vi "Save_to_Project.vi"(8 "error in (no error)":errorcluster, 9 "index in":string, 10 "buildObject":T1, 11 "Class in":refnum<class "IB_Source_Container.lvclass">) -> (0 "error out":errorcluster, 1 "index out":string, 2 "buildObject out":T1, 3 "Class out":refnum<class "IB_Source_Container.lvclass">, 5 "saved?":bool)   [LabVIEW 2020, in "IB_Source_Container.lvclass"]
uses:
  <vilib>/AppBuilder/IB_Classes/Source/Container/IB_Source_Container.lvclass
  <vilib>/AppBuilder/IB_Classes/Source/Container/IB_Source_Container.lvclass/IB_Source_Container.ctl
  <vilib>/AppBuilder/IB_Classes/Source/IB_Source.lvclass
  <vilib>/AppBuilder/IB_Classes/Source/File/CtrFile/IB_CtrFile.lvclass
  <resource>/Framework/Providers/API/ItemRef.ctl
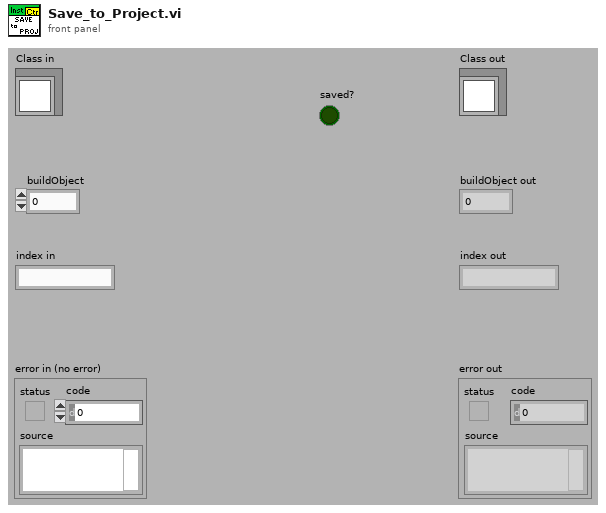
[diagram p1: front panel]
types:
  T1 = typedef "ItemRef.ctl" = u64
  T2 = typedef "IB_CtrFile.ctl" = cluster{"parentTag":string, "force save?":bool}
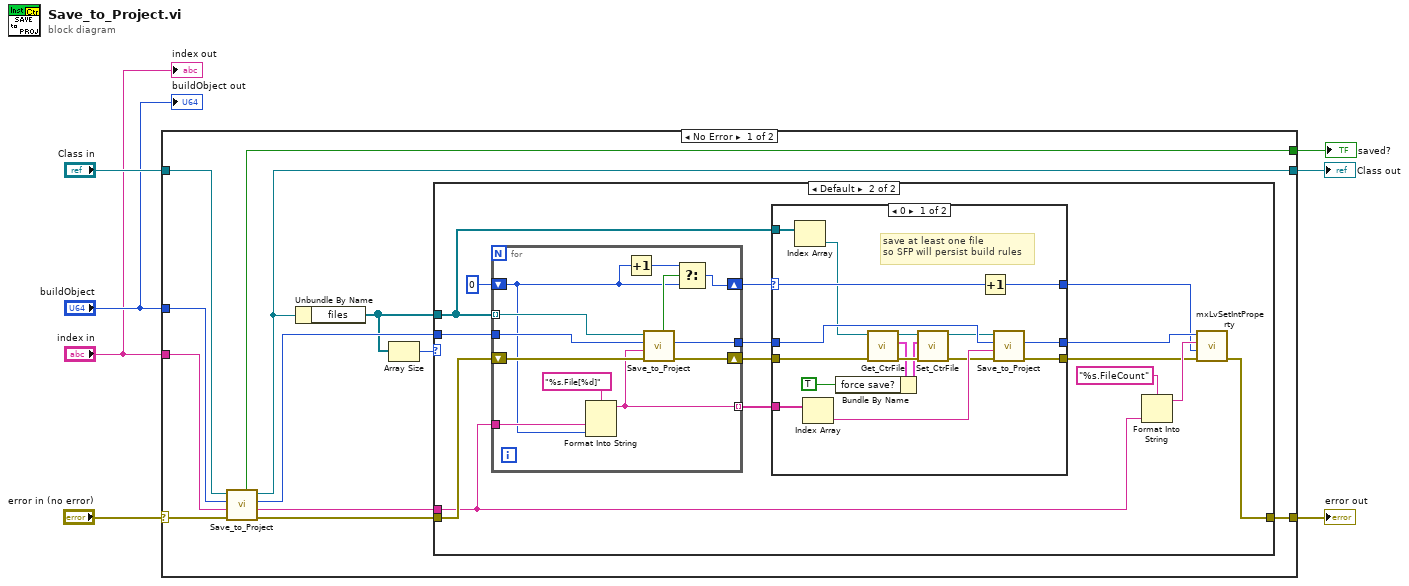
[diagram p0: block diagram]
diagram:
  n1 = case shown="No Error" "error in (no error)" {
    selector: "error in (no error)" -> [w16 w69]
    tunnel: [w9 w69] -> w7
    tunnel: [w15 w68] -> w6
    tunnel: "index in" -> [w19 _]
    tunnel: "buildObject" -> [w18 _]
    tunnel: "Class in" -> [w17 w68]
    tunnel: [w8 _] -> w1
    frame No Error {
      n2 = call-parent "Save_to_Project.vi"("error in (no error)"=w16, "index in"=w19, "buildObject"=w18, "Class in"=w17) -> ("error out"=w10:errorcluster, "index out"=w12:string, "buildObject out"=w14:T1, "Class out"=w15:refnum<class "IB_Source_Container.lvclass">, "saved?"=w8:bool)  [unwired: 3 out]
      n3 = Unbundle By Name(w15) -> ("files"=w13:refnum<class "IB_CtrFile.lvclass">[])
      n4 = Array Size(array=w13) -> (size(s)=w11:i32)
      n5 = case shown="Default" w11 {
        tunnel: w14 -> [_ w35]
        tunnel: w13 -> [_ w23]
        tunnel: w12 -> [_ w22]
        tunnel: w10 -> [w20 w33]
        tunnel: [w20 w27] -> w9
        frame 0 {
        }
        frame Default {
          n6 = for {
            tunnel: w23 -> [w67] mode=indexing
            tunnel: w35 -> [w66]
            tunnel: w22 -> [w64]
            shift-right: [w63] -> w34
            shift-left: w33 -> [w62]
            tunnel: [w61] -> w26
            shift-right: [w59] -> w31
            shift-left: 0 -> [w57]
            tunnel: [w56] -> w21 mode=indexing
            n7 = Format Into String(format string="%s.File[%d]", w64, w57) -> (resulting string=w56:string)  [unwired: 2 in, 1 out]
            n8 = Increment(x=w57) -> (x+1=w60:i32)
            n9 = call-dynamic "Save_to_Project.vi"("error in (no error)"=w62, "index in"=w56, "buildObject"=w66, "Class in"=w67) -> ("error out"=w63:errorcluster, "buildObject out"=w61:T1, "saved?"=w58:bool)  [unwired: 5 out]
            n10 = Select(t=w60, s=w58, f=w57) -> (s? t:f=w59:i32)
          }
          n11 = case shown="0" w31 {
            selector: w31 -> [w51 w53]
            tunnel: w34 -> [w40 w55]
            tunnel: [w52 w55] -> w28
            tunnel: w26 -> [w50 w54]
            tunnel: [w49 w54] -> w25
            tunnel: [w48 w53] -> w24
            tunnel: w23 -> [w47 _]
            tunnel: w21 -> [w46 _]
            frame 0 {
              # "save at least one file\nso SFP will persist build rules"
              n12 = Index Array(array=w47) -> (element=w42:refnum<class "IB_CtrFile.lvclass">)  [unwired: 1 in]
              n13 = Index Array(array=w46) -> (element=w45:string)  [unwired: 1 in]
              n14 = call <vilib>:"Get_CtrFile.vi"("error in (no error)"=w40, "IB_CtrFile in"=w42) -> ("error out"=w44:errorcluster, "parentTag"=w38:T2, "IB_CtrFile out"=w43:refnum<class "IB_CtrFile.lvclass">)  [unwired: 7 out]
              n15 = Bundle By Name(cluster=w38, "force save?"=TRUE) -> (w37:T2)
              n16 = call <vilib>:"Set_CtrFile.vi"("error in (no error)"=w44, "parentTag"=w37, "IB_CtrFile in"=w43) -> ("error out"=w39:errorcluster, "IB_CtrFile out"=w41:refnum<class "IB_CtrFile.lvclass">)  [unwired: 7 out]
              n17 = Increment(x=w51) -> (x+1=w48:i32)
              n18 = call-dynamic "Save_to_Project.vi"("error in (no error)"=w39, "index in"=w45, "buildObject"=w50, "Class in"=w41) -> ("error out"=w52:errorcluster, "buildObject out"=w49:T1)  [unwired: 6 out]
            }
            frame Default {
            }
          }
          n19 = Format Into String(format string="%s.FileCount", w22) -> (resulting string=w30:string)  [unwired: 2 in, 1 out]
          n20 = call <resource>:"mxLvSetIntProperty.vi"("error in"=w28, "Value (0)"=w24, "Tag"=w30, "Item"=w25) -> ("error out"=w27:errorcluster)  [unwired: 1 in, 6 out]
        }
      }
    }
    frame Error {
    }
  }
  "error out" <- w7
  "Class out" <- w6
  "saved?" <- w1
  "buildObject out" <- "buildObject"
  "index out" <- "index in"
